vi "ReadDevicesList.vi"(8 "error in":errorcluster, 10 "delimiter of string answer (semicolon)":string=";", 11 "JSON":string="{}") -> (0 "error out":errorcluster, 2 "table of devices":string[][](array[string]), 3 "unformated list of devices":string[](array[string]))   [LabVIEW 2023, in "DeviceManager.lvlib"]
uses:
  DeviceManager.lvlib
  b7523fc8-2a53-440f-95db-1f4af3dd9b6b.vi
  <vilib>/JDP Science/JSONtext/Find Item.vi
  <vilib>/JDP Science/JSONtext/Next JSON Value.vi
  <vilib>/JDP Science/JSONtext/String Subset.vi
  <vilib>/JDP Science/JSONtext/Parsing/Advance past next JSON Value (inlined COPY).vi
  <vilib>/JDP Science/JSONtext/Parsing/Advance past whitespace.vi
  <vilib>/JDP Science/JSONtext/Parsing/Advance past String.vi
  <vilib>/JDP Science/JSONtext/Parsing/Advance past Number.vi
  <vilib>/JDP Science/JSONtext/Parsing/Advance past Line Ending.vi
  <vilib>/JDP Science/JSONtext/Parsing/Parse Full Path or Item Name.vi
  <vilib>/JDP Science/JSONtext/Parsing/Advance past Array.vi
  <vilib>/JDP Science/JSONtext/Parsing/Advance past Object.vi
  <vilib>/JDP Science/JSONtext/support/Error Cluster From Code.vi
  <vilib>/JDP Science/JSONtext/Offset/Find Item Locations by Path.vi
  <vilib>/JDP Science/JSONtext/JSON text to Variant.vi
  <vilib>/JDP Science/JSONtext/LVClass Serializer/JSONtext LVClass Serializer.lvclass
panel:
  # "Connector Pane"
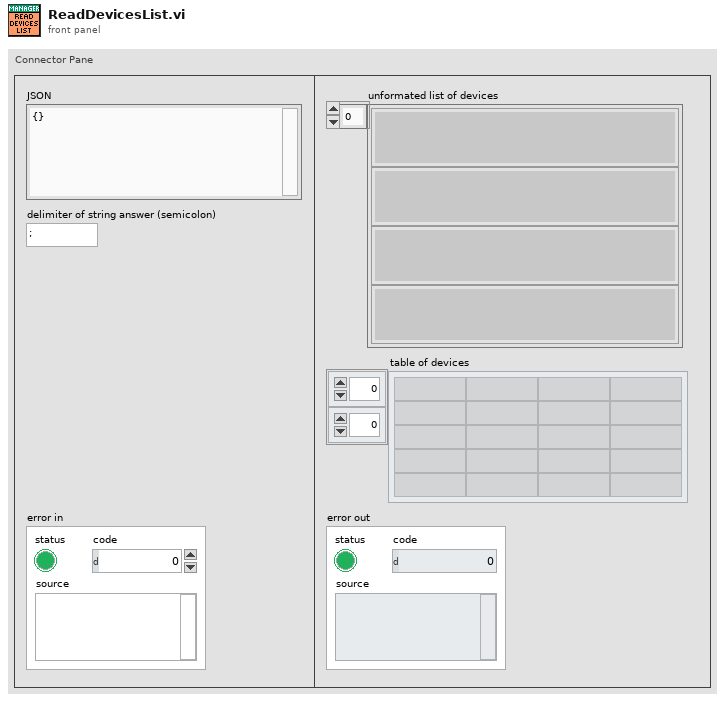
[diagram p1: front panel]
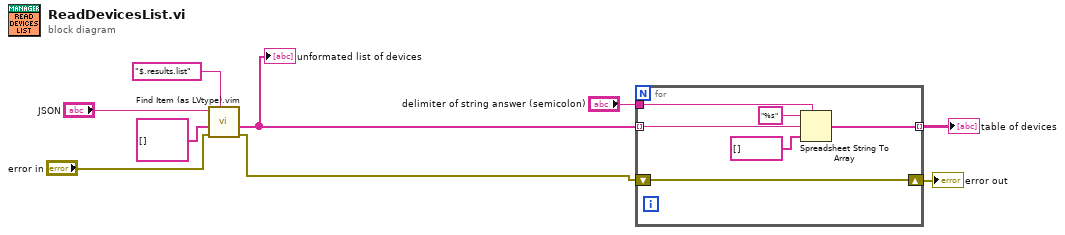
[diagram p0: block diagram]
diagram:
  n1 = call "Find Item (as LVtype).vim"("$Path or Item Name"="$.results.list" ("Label (VI Title)"), "error in (no error)"="error in", "Data Type and Default Value"=string[] [], "JSON"="JSON") -> ("error out"=w2:errorcluster, "Data"=w5:string[])  [unwired: 4 in, 2 out]
  "unformated list of devices" <- w5
  n2 = for {
    tunnel: w5 -> [w12] mode=indexing
    tunnel: [w13] -> w4 mode=indexing
    tunnel: "delimiter of string answer (semicolon)" -> [w11]
    shift-right: [w10] -> w1
    shift-left: w2 -> [w10]
    n3 = Spreadsheet String To Array(delimiter (Tab)=w11, format string="%s", spreadsheet string=w12, array type (2D Dbl)=string[] []) -> (array=w13:string[])
  }
  "table of devices" <- w4
  "error out" <- w1
